vi "sensorCheck.vi"(6 "Temp Button Press":bool, 7 "Endgame yet?":bool, 8 "Sensor Margin of Error":dbl, 9 "Acceptable Distance":dbl, 10 "Right Sensor Value":dbl, 11 "Left Sensor Value":dbl) -> (3 "In range":bool)   [LabVIEW 2018]
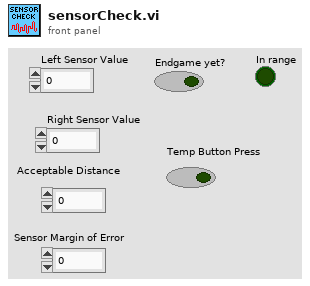
[diagram p1: front panel]
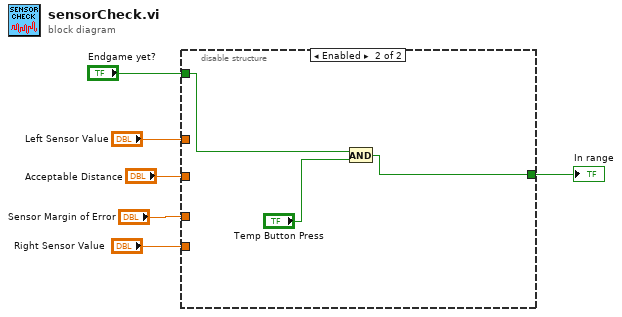
[diagram p0: block diagram]
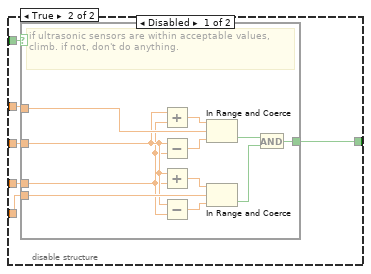
[diagram p2: hidden frame]
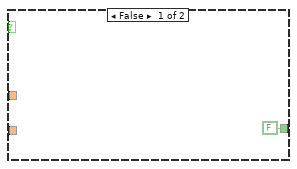
[diagram p3: hidden frame]
diagram:
  n1 = disable-structure shown="Enabled" {
    disable-tunnel: "Sensor Margin of Error" -> [w12 _]
    disable-tunnel: "Acceptable Distance" -> [w11 _]
    disable-tunnel: "Left Sensor Value" -> [w10 _]
    disable-tunnel: "Right Sensor Value" -> [w9 _]
    disable-tunnel: "Endgame yet?" -> [w8 w27]
    disable-tunnel: [w7 w25] -> w1
    frame Disabled {
      n2 = case shown="True" w8 {
        tunnel: w12 -> [_ w17]
        tunnel: w11 -> [_ w18]
        tunnel: w9 -> [_ w19]
        tunnel: w10 -> [_ w22]
        tunnel: [FALSE w14] -> w7
        frame False {
        }
        frame True {
          # "if ultrasonic sensors are within acceptable values, climb. if not, don't do anything."
          n3 = Add(x=w18, y=w17) -> (x+y=w24:dbl)
          n4 = Subtract(x=w18, y=w17) -> (x-y=w23:dbl)
          n5 = Add(x=w18, y=w17) -> (x+y=w20:dbl)
          n6 = Subtract(x=w18, y=w17) -> (x-y=w21:dbl)
          n7 = In Range and Coerce(upper limit=w24, x=w22, lower limit=w23) -> (In Range?=w16:bool)  [unwired: 1 out]
          n8 = In Range and Coerce(upper limit=w20, x=w19, lower limit=w21) -> (In Range?=w15:bool)  [unwired: 1 out]
          n9 = And(x=w16, y=w15) -> (x .and. y?=w14:bool)
        }
      }
    }
    frame Enabled {
      n10 = And(x=w27, y="Temp Button Press") -> (x .and. y?=w25:bool)
    }
  }
  "In range" <- w1
